vi "Activate PAS Board.vi"(8 "error in (no error)":errorcluster) -> (0 "error out":errorcluster, 3 "Session Handle out":T1 caption="Gas")   [LabVIEW 2015, in "PAS.lvclass"]
uses:
  PAS.lvclass
  Typedefs/Session Handle.ctl
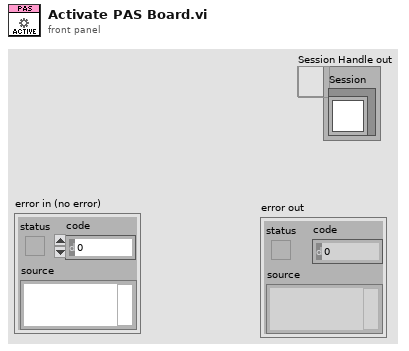
[diagram p1: front panel]
types:
  T1 = typedef "PAS.lvclass/Session Handle.ctl" = refnum<data-value>
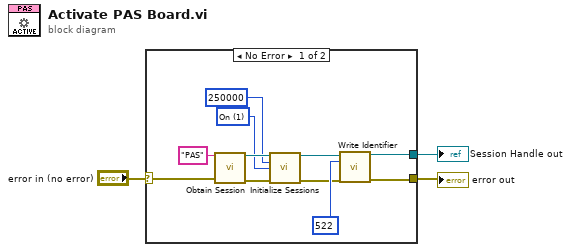
[diagram p0: block diagram]
diagram:
  n1 = case shown="No Error" "error in (no error)" {
    selector: "error in (no error)" -> [w8 w15]
    tunnel: [w5 w15] -> w3
    tunnel: [w4 _] -> w1
    frame No Error {
      w11 = u32 1 items=["Off", "On"] ("Termination")
      n2 = call "Obtain Session.vi"("Session  Name ()"="PAS", "error in (no error)"=w8) -> ("Session Handle"=w13:T1, "error out"=w14:errorcluster)  [unwired: 12 in]
      n3 = call "Initialize Sessions.vi"("Session Handle in"=w13, "Baud Rate"=u32 250000, "Termination"=w11, "error in (no error)"=w14) -> ("Session Handle Out"=w6:T1, "error out"=w7:errorcluster)  [unwired: 10 in]
      n4 = call "Write Identifier.vi"("Session Handle in"=w6, "identifier"=u16 522, "error in (no error)"=w7) -> ("Session Handle out"=w4:T1, "error out"=w5:errorcluster)  [unwired: 11 in]
    }
    frame Error {
    }
  }
  "error out" <- w3
  "Session Handle out" <- w1
